vi "HFRR ADV v036.vi"() -> ()   [LabVIEW 2025] (continued)
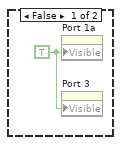
[diagram p5: hidden frame]
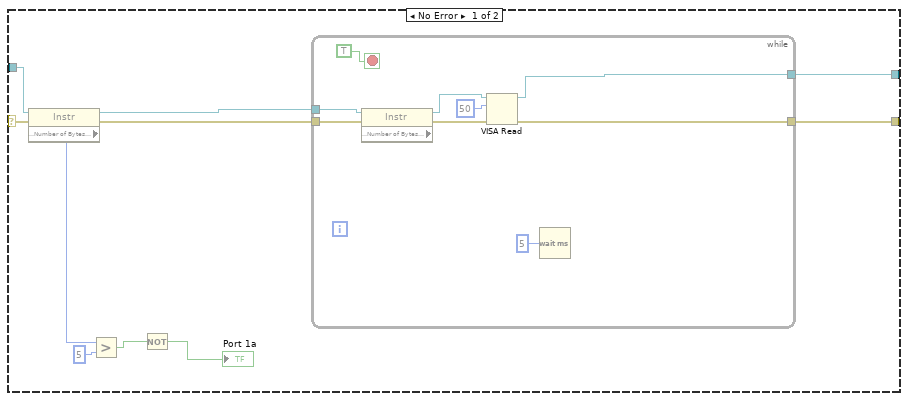
[diagram p6: hidden frame]
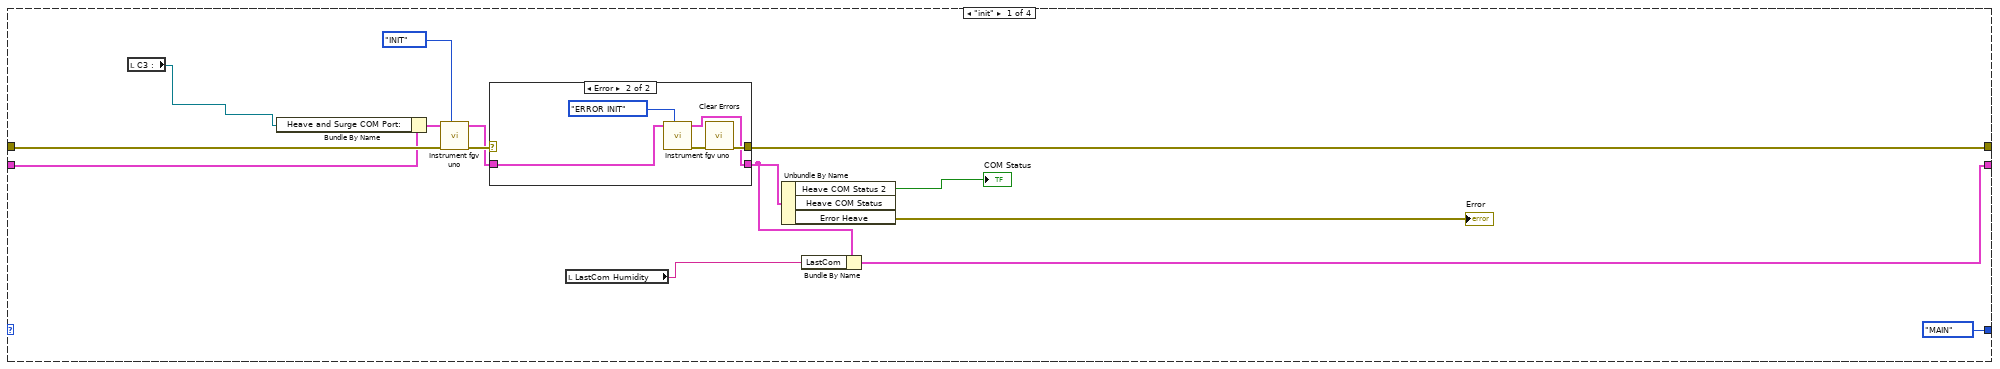
[diagram p8: hidden frame]
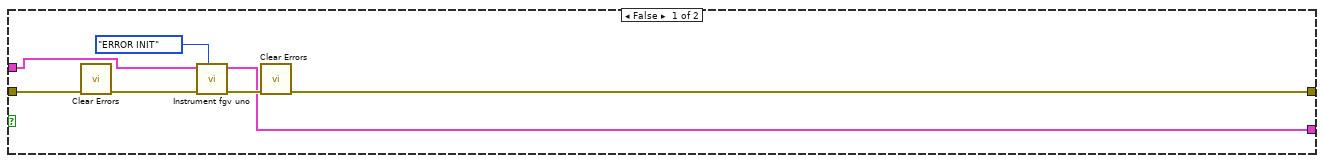
[diagram p10: hidden frame]
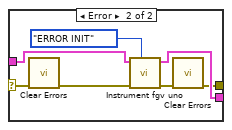
[diagram p12: hidden frame]
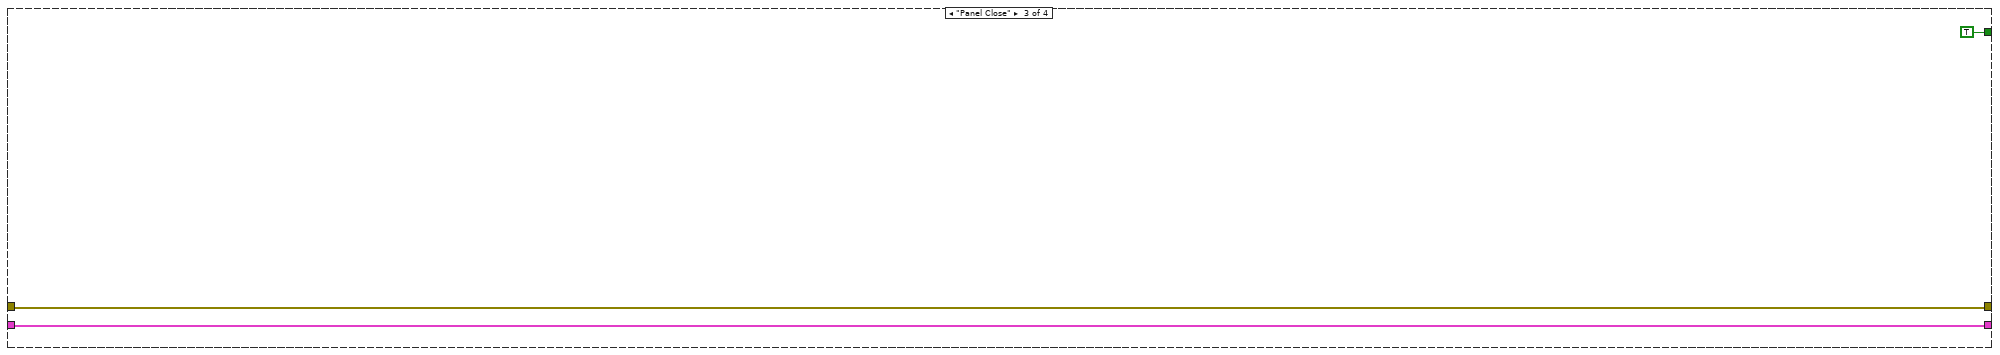
[diagram p14: hidden frame]
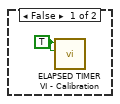
[diagram p18: hidden frame]
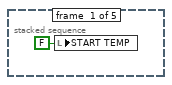
[diagram p20: hidden frame]
        n3362 = Equal?(x=w4392, y=0.0) -> (x = y?=w4394:bool)
        n3363 = case shown="True" w4394 {
          tunnel: [w4415 w4416] -> w4393
          tunnel: w4392 -> [w4415 _]
          frame False {
            (unwired) 0.0
            "Humidity temp" <- w4415
          }
          frame True {
            n3364 = local read "Humidity temp"() -> (w4416:dbl)
          }
        }
        "RH Numeric:" <- w4393
      }
      frame Enabled {
        n3365 = local read "Read HUMIDITY"() -> (w4440:string)
        n3366 = Spreadsheet String To Array(delimiter (Tab)=",", format string="", spreadsheet string=w4440, array type (2D Dbl)=dbl[] []) -> (array=w4436:dbl[])
        n3367 = Index Array(array=w4436) -> (element #1=→"STATE :":dbl, element #2=→"SET :":dbl, element #3=w4420:dbl, element #4=→"RH :":dbl, element #5=→"T :":dbl, element #6=→"AMB_RH :":dbl, element #7=→"AMB_T :":dbl, element #8=→"PUMP :":dbl, element #9=→"FAN_IN :":dbl, element #10=→"FAN_OUT :":dbl, element #11=→"DEHUM :":dbl, element #12=→"CURRENT :":dbl, element #13=→"STALL":dbl)  [unwired: 13 in]
        "RH Numeric:" <- w4420
        n3368 = Equal?(x=w4420, y=0.0) -> (x = y?=w4423:bool)
        n3369 = case shown="False" w4423 {
          tunnel: [w4441 w4442] -> w4424
          tunnel: w4420 -> [w4441 _]
          frame False {
            "Humidity temp 2" <- w4441
          }
          frame True {
            n3370 = local read "Humidity temp 2"() -> (w4442:dbl)
          }
        }
        n3371 = local write "RH Numeric:"(w4424) -> ()
      }
    }
    n3372 = local read "Quit"() -> (w4390:bool)
  }
  n3373 = while {
    shift-right: [w4448] -> _
    shift-left: _ -> [w4449]
    shift-right: [w4446] -> _
    shift-left: T20 {"Read Uno"="", "Bytes at Heave Port"=0.0, "UNO COM Port:"="COM9", "UNO COM Port: 2"="COM7", "Residual Due"="", "UNO COM Status 2"=TRUE, "UNO COM Status"=TRUE, "Port 2"=TRUE, "Sway PPR"=6400.0, "Surge PPR"=6400.0, "Heave PPR"=6400.0, "Sway Pitch"=2.0, "Surge Pitch"=3.0, "Heave Pitch"=4.0, "Sway Pulses/mm"=320.0, "Surge Pulses/mm"=1600.0, "Heave Pulses/mm"=1600.0, "inner loop"=0.0, "Read Heave and Surge 2"="", "String 36"="", "Write S"=FALSE, "WriteCC1"=[""], "Heave COM Loop"=0, "LastCom"="", "EXIT"=FALSE, "Error Heave"={"status"=TRUE, "code"=-1073807343, "source"=""}} -> [w4445]
    shift-right: [w4443] -> _
    shift-left: enum16{"init", "MAIN", "Panel Close"}."init" -> [w4444]
    stop <- w4447 stop-if-true
    # "UNO CODE LOGIC"
    n3374 = case shown="\"MAIN\"" w4444 {
      tunnel: w4449 -> [w4463 w4482 w4538 w4540]
      tunnel: [w4458 w4487 w4538 w4540] -> w4448
      tunnel: [_ _ TRUE _] -> w4447
      tunnel: [w4454 w4485 w4536 w4539] -> w4446
      tunnel: w4445 -> [w4460 w4481 w4536 w4539]
      tunnel: [enum16{"init", "MAIN", "Panel Close"}."MAIN" w4476 _ _] -> w4443
      frame "init" {
        n3375 = local read "Com Port 1"() -> (w4450:refnum<visa-resource-name>)
        n3376 = Bundle By Name(cluster=w4460, "UNO COM Port:"=w4450) -> (w4459:T20)
        n3377 = call "Instrument fgv.vi"("Enum"=T32."INIT", "error in (no error) 2"=w4463, "INPUT"=w4459) -> ("error"=w4461:errorcluster, "output"=w4457:T18)  [unwired: 6 in, 1 out]
        n3378 = case shown="Error" w4461 {
          selector: w4461 -> [w4465 _]
          tunnel: [w4465 w4469] -> w4458
          tunnel: w4457 -> [w4464 w4467]
          tunnel: [w4464 w4466] -> w4455
          frame No Error {
          }
          frame Error {
            n3379 = call "Instrument fgv.vi"("Enum"=T32."ERROR INIT", "INPUT"=w4467) -> ("error"=w4470:errorcluster, "output"=w4466:T18)  [unwired: 7 in, 1 out]
            n3380 = call <vilib>:"Clear Errors.vi"("error in (no error)"=w4470) -> ("error out"=w4469:errorcluster)  [unwired: 5 in, 1 out]
          }
        }
        n3381 = local read "LastCom UNO"() -> (w4452:string)
        n3382 = Unbundle By Name(w4455) -> ("Heave COM Status 2"=→"Instrument Status":bool, "Error Heave"=→"Error  2":errorcluster)  [unwired: 1 out]
        n3383 = Bundle By Name(cluster=w4455, "LastCom"=w4452) -> (w4454:T18)
      }
      frame "MAIN" {
        n3384 = Unbundle By Name(w4481) -> ("UNO COM Port: 2"=w4471:refnum<visa-resource-name>)
        n3385 = local read "Com Port 1"() -> (w4472:refnum<visa-resource-name>)
        n3386 = local write "COM Port UNO :"(w4471) -> ()
        n3387 = Equal?(x=w4471, y=w4472) -> (x = y?=w4488:bool)
        n3388 = Bundle By Name(cluster=w4481, "UNO COM Port:"=w4472) -> (w4480:T20)
        n3389 = case shown="True" w4488 {
          tunnel: [w4492 w4509] -> w4487
          tunnel: w4482 -> [w4493 w4515]
          tunnel: w4480 -> [w4491 w4513]
          tunnel: [w4490 w4508] -> w4485
          frame False {
            n3390 = call <vilib>:"Clear Errors.vi"("error in (no error)"=w4493) -> ("error out"=w4489:errorcluster)  [unwired: 5 in, 1 out]
            n3391 = call "Instrument fgv.vi"("Enum"=T32."ERROR INIT", "error in (no error) 2"=w4489, "INPUT"=w4491) -> ("error"=w4495:errorcluster, "output"=w4490:T18)  [unwired: 6 in, 1 out]
            n3392 = call <vilib>:"Clear Errors.vi"("error in (no error)"=w4495) -> ("error out"=w4492:errorcluster)  [unwired: 5 in, 1 out]
          }
          frame True {
            n3393 = call "Instrument fgv.vi"("Enum"=T32."READ", "error in (no error) 2"=w4515, "INPUT"=w4513) -> ("error"=w4514:errorcluster, "output"=w4507:T18)  [unwired: 6 in, 1 out]
            n3394 = Bundle By Name(cluster=w4507, "String 36"="WRITE UNO") -> (w4506:T18)
            n3395 = case shown="True" "Write" {
              selector: "Write" -> [_ w4530]
              tunnel: w4514 -> [w4528 w4535]
              tunnel: [w4528 w4534] -> w4504
              tunnel: w4506 -> [w4527 w4532]
              tunnel: [w4527 w4531] -> w4503
              frame False {
              }
              frame True {
                n3396 = Not(x=w4530) -> (.not. x?=w4529:bool)
                n3397 = local write "Write"(w4529) -> ()
                n3398 = call "Instrument fgv.vi"("Enum"=T32."MANUAL WRITE", "error in (no error) 2"=w4535, "INPUT"=w4532) -> ("error"=w4534:errorcluster, "output"=w4531:T18)  [unwired: 6 in, 1 out]
              }
            }
            n3399 = Array Size(array="Write UNO") -> (size(s)=w4501:i32)
            n3400 = Greater Than 0?(x=w4501) -> (x > 0?=w4500:bool)
            n3401 = call "Instrument fgv.vi"("Enum"=T32."WRITE", "error in (no error) 2"=w4504, "WriteCC1"="Write UNO", "INPUT"=w4503) -> ("error"=w4511:errorcluster, "WriteCC1 2"=w4502:string[], "output"=w4510:T18)  [unwired: 5 in]
            n3402 = case shown="True" w4500 {
              tunnel: w4502 -> [_ w4517]
              frame False {
              }
              frame True {
                n3403 = local write "Write UNO"(w4517) -> ()
              }
            }
            n3404 = case shown="Error" w4511 {
              selector: w4511 -> [w4518 w4521]
              tunnel: w4510 -> [w4519 w4526]
              tunnel: [w4519 w4525] -> w4508
              tunnel: [w4518 w4523] -> w4509
              frame No Error {
              }
              frame Error {
                n3405 = call <vilib>:"Clear Errors.vi"("error in (no error)"=w4521) -> ("error out"=w4520:errorcluster)  [unwired: 5 in, 1 out]
                n3406 = call "Instrument fgv.vi"("Enum"=T32."ERROR INIT", "error in (no error) 2"=w4520, "INPUT"=w4526) -> ("error"=w4524:errorcluster, "output"=w4525:T18)  [unwired: 6 in, 1 out]
                n3407 = call <vilib>:"Clear Errors.vi"("error in (no error)"=w4524) -> ("error out"=w4523:errorcluster)  [unwired: 5 in, 1 out]
              }
            }
            n3408 = Unbundle By Name(w4508) -> ("LastCom"=→"LastCom UNO":string, "Read Heave and Surge"=→"Read UNO":string)
          }
        }
        n3409 = Unbundle By Name(w4485) -> ("Heave COM Status 2"=w4486:bool, "Heave COM Status"=w4475:bool, "Error Heave"=w4473:errorcluster, "Bytes at Heave Port"=→"Bytes at Humidity Port":dbl)
        n3410 = Not(x=w4475) -> (.not. x?=w4483:bool)
        n3411 = Not(x=w4486) -> (.not. x?=w4474:bool)
        n3412 = local write "Instrument Status"(w4483) -> ()
        n3413 = local write "Error  2"(w4473) -> ()
        n3414 = local write "Port 1a"(w4475) -> ()
        n3415 = local read "Quit"() -> (w4477:bool)
        n3416 = local write "COM Status"(w4474) -> ()
        n3417 = Select(t=enum16{"init", "MAIN", "Panel Close"}."Panel Close", s=w4477, f=enum16{"init", "MAIN", "Panel Close"}."MAIN") -> (s? t:f=w4476:enum16{"init", "MAIN", "Panel Close"})
      }
      frame "Panel Close" {
      }
      frame Default {
      }
    }
  }
